vi "Split byte.vi"(10 "Value":dbl=1000.0) -> (2 "Array":dbl[](array[numeric]))   [LabVIEW 2010, in "Yudian AI508.lvlib"]
uses:
  <instrlib>/Yudian AI508/Yudian AI508.lvlib
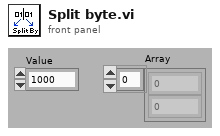
[diagram p1: front panel]
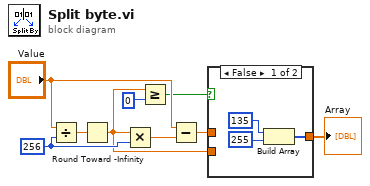
[diagram p0: block diagram]
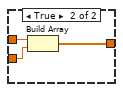
[diagram p2: hidden frame]
diagram:
  w8 = 256
  n1 = Divide(x="Value", y=w8) -> (x/y=w9:dbl)
  n2 = Round Toward -Infinity(1:w9) -> (0:w3:dbl)
  n3 = Multiply(x=w3, y=w8) -> (x*y=w6:dbl)
  n4 = Greater Or Equal?(x=w3, y=0) -> (x >= y?=w2:bool)
  n5 = Subtract(x="Value", y=w6) -> (x-y=w7:dbl)
  n6 = case shown="False" w2 {
    tunnel: w7 -> [_ w15]
    tunnel: w3 -> [_ w14]
    tunnel: [w10 w13] -> w1
    frame False {
      n7 = Build Array(135, 255) -> (w10:i32[])
    }
    frame True {
      n8 = Build Array(w15, w14) -> (w13:dbl[])
    }
  }
  "Array" <- w1
